vi "加载数据.vi"(11 "数据路径":path caption="文件路径 （空时为对话框）") -> (2 "数据":cluster{dbl[], dbl[]}[](graph), 3 "数据名称":string[](array[string]))   [LabVIEW 2019]
uses:
  <vilib>/Utility/file.llb/Read Delimited Spreadsheet (string).vi
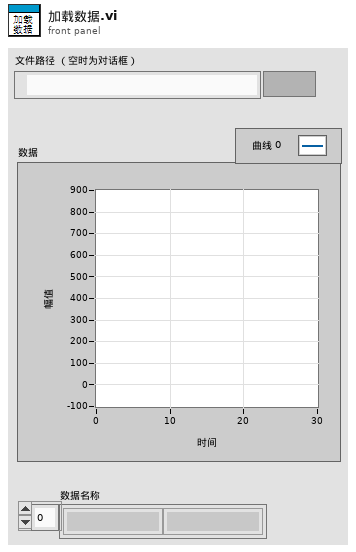
[diagram p1: front panel]
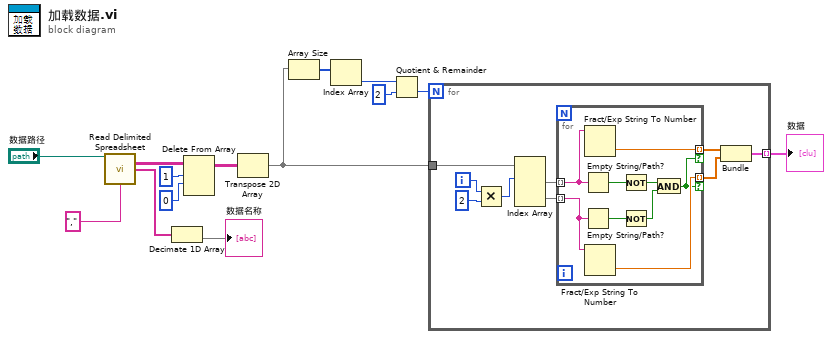
[diagram p0: block diagram]
diagram:
  n1 = call-poly <vilib>:"Read Delimited Spreadsheet.vi"("file path (dialog if empty)"="数据路径", "delimiter (\\t)"="," ("delimiter (\\t)")) -> ("all rows"=w12:string[][], "first row"=w2:string[])  [unwired: 8 in, 4 out]
  n2 = Decimate 1D Array(w2) -> (→"数据名称":string[])  [unwired: 1 out]
  n3 = Delete From Array(array=w12, length=1 ("长度"), index (row)=0 ("索引 (行)")) -> (array with subset deleted=w9:string[][])  [unwired: 1 in, 1 out]
  n4 = Transpose 2D Array(2D array=w9) -> (transposed array=w8:string[][])
  n5 = Array Size(array=w8) -> (size(s)=w7:i32[])
  n6 = Index Array(array=w7) -> (element=w6:i32)  [unwired: 1 in]
  n7 = Quotient & Remainder(x=w6, y=2) -> (floor(x/y)=w4:i32)  [unwired: 1 out]
  n8 = for {
    N: w4 -> [_]
    tunnel: w8 -> [w23]
    tunnel: [w19] -> w3 mode=indexing
    i -> [w20]
    n9 = Multiply(x=w20, y=2) -> (x*y=w21:i32)
    n10 = Index Array(array=w23, index (row) #1=w21) -> (element #1=w16:string[], element #2=w18:string[])  [unwired: 3 in]
    n11 = for {
      tunnel: [w32] -> w15 mode=indexing if=w25
      tunnel: w18 -> [w27] mode=indexing
      tunnel: [w31] -> w17 mode=indexing if=w25
      tunnel: w16 -> [w30] mode=indexing
      n12 = Empty String/Path?(string/path=w30) -> (empty?=w29:bool)
      n13 = Empty String/Path?(string/path=w27) -> (empty?=w26:bool)
      n14 = Fract/Exp String To Number(string=w30) -> (number=w32:dbl)  [unwired: 3 in, 1 out]
      n15 = Fract/Exp String To Number(string=w27) -> (number=w31:dbl)  [unwired: 3 in, 1 out]
      n16 = Not(x=w29) -> (.not. x?=w28:bool)
      n17 = Not(x=w26) -> (.not. x?=w24:bool)
      n18 = And(x=w28, y=w24) -> (x .and. y?=w25:bool)
    }
    n19 = Bundle(w15, w17) -> (w19:cluster{dbl[], dbl[]})  [unwired: 1 in]
  }
  "数据" <- w3
